vi "Locate.vi"() -> ()   [LabVIEW 2017]
uses:
  <vilib>/Utility/file.llb/Write Delimited Spreadsheet (DBL).vi
  <vilib>/vision/driver/NI_Vision_Acquisition_Software.lvlib
  <vilib>/vision/NI_Vision_Development_Module.lvlib
panel:
  out "Boolean 2":bool
  out "X":dbl[](array[numeric])
  out "Numeric 2":dbl
  out "Numeric":dbl
  out "OK Y":dbl
  out "OK X":dbl
  in  "OK Button":bool
  out "Boolean":bool
  out "Y":dbl[](array[numeric])
  out "選擇範圍 2":T1(plugin-control)
  out "error out":errorcluster
  in  "亮度":cluster{"Min":i32, "Max":i32}(slide)={"Min"=60, "Max"=157} scale=0.0..255.0
  in  "飽和度":cluster{"Min":i32, "Max":i32}(slide)={"Min"=0, "Max"=42} scale=0.0..255.0
  in  "色相":cluster{"Min":i32, "Max":i32}(slide)={"Min"=67, "Max"=120} scale=0.0..255.0
  out "顯示錯誤":errorcluster
  out "影像":T1(plugin-control)
  in  "stop":bool
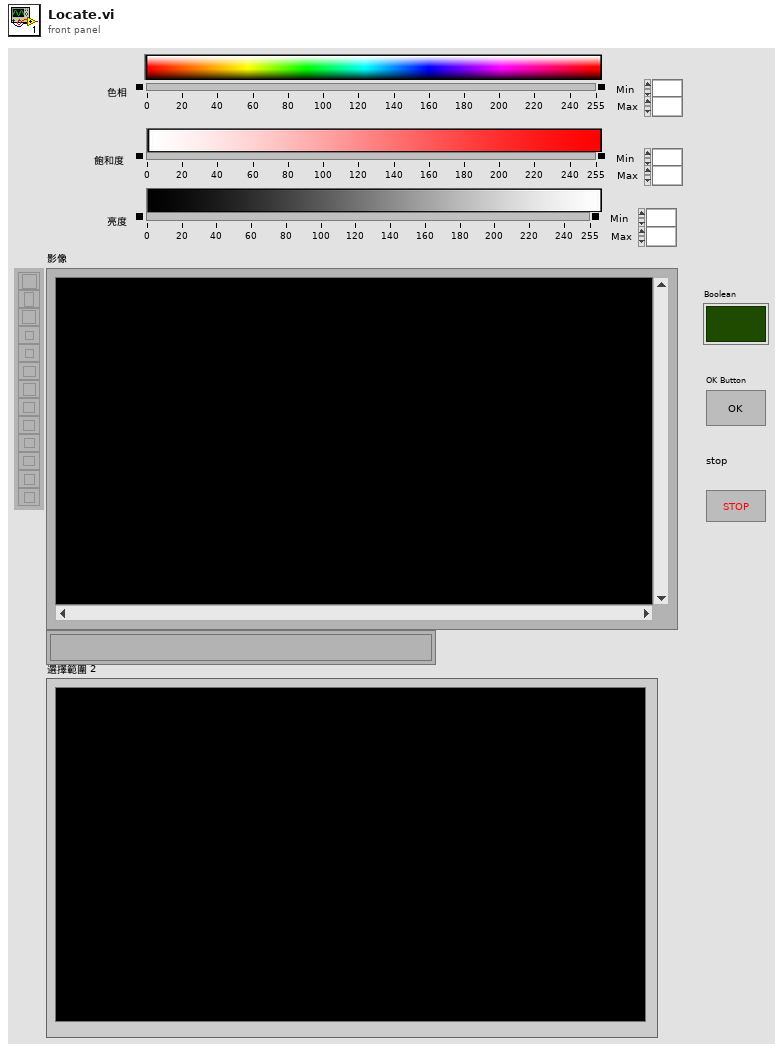
[diagram p1: front panel]
types:
  T1 = typedef "IMAQ Image.ctl" = refnum<image>
  T2 = typedef "Image Type" = u32
  T3 = cluster{"Type":u32, "Version":u32, "Flags":u32, "SerialNumberHigh":u32, "SerialNumberLow":u32, "BusType":u32, "InterfaceName":string, "VendorName":string, "ModelName":string, "CameraFileName":string, "CameraAttributeURL":string}[]
  T4 = cluster{"Type":u32, "Version":u32, "Flags":u32, "SerialNumberHigh":u32, "SerialNumberLow":u32, "BusType":u32, "InterfaceName":string, "VendorName":string, "ModelName":string, "CameraFileName":string, "CameraAttributeURL":string}
  T5 = typedef "IMAQdx.ctl" = refnum<k21>
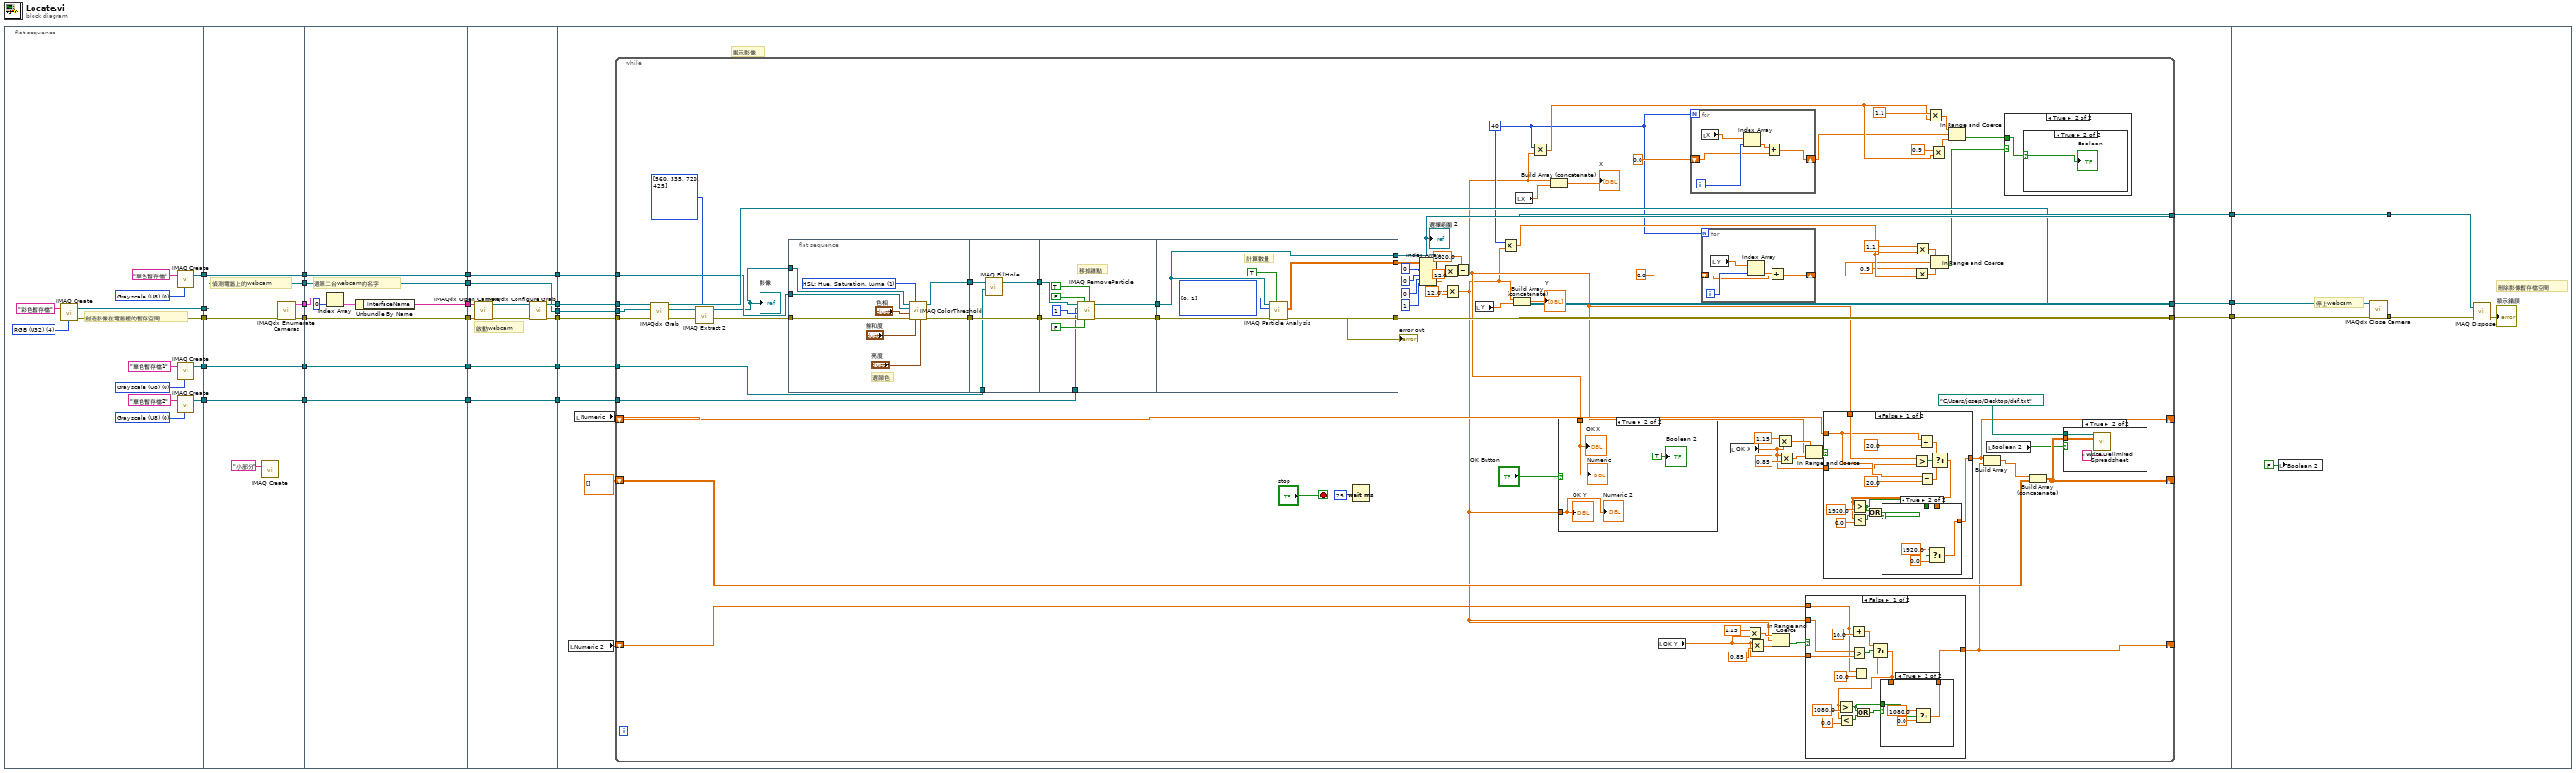
[diagram p0: block diagram]
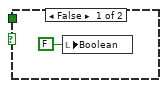
[diagram p3: hidden frame]
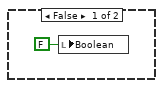
[diagram p4: hidden frame]
diagram:
  n1 = flat-sequence {
    tunnel: [w39] -> w22
    tunnel: [w38] -> w21
    tunnel: [w35] -> w12
    tunnel: [w30] -> w5
    tunnel: [w29] -> w1
    tunnel: [w49] -> w28
    tunnel: [w48] -> w23
    tunnel: w22 -> [w48]
    tunnel: w21 -> [w47]
    tunnel: [w46] -> w19
    tunnel: [w45] -> w13
    tunnel: w12 -> [w45]
    tunnel: [w44] -> w6
    tunnel: w5 -> [w44]
    tunnel: [w43] -> w2
    tunnel: w1 -> [w43]
    tunnel: w28 -> [w56]
    tunnel: [w55] -> w27
    tunnel: [w54] -> w24
    tunnel: w23 -> [w54]
    tunnel: [w53] -> w20
    tunnel: w19 -> [w53]
    tunnel: [w52] -> w14
    tunnel: w13 -> [w52]
    tunnel: [w51] -> w7
    tunnel: w6 -> [w51]
    tunnel: [w50] -> w3
    tunnel: w2 -> [w50]
    tunnel: w27 -> [w67]
    tunnel: [w66] -> w26
    tunnel: [w65] -> w25
    tunnel: w24 -> [w65]
    tunnel: w20 -> [w64]
    tunnel: [w62] -> w18
    tunnel: [w61] -> w15
    tunnel: w14 -> [w61]
    tunnel: [w60] -> w8
    tunnel: w7 -> [w60]
    tunnel: [w59] -> w4
    tunnel: w3 -> [w59]
    tunnel: w26 -> [w80]
    tunnel: w25 -> [w79]
    tunnel: w18 -> [w78]
    tunnel: [w77] -> w16
    tunnel: w15 -> [w76]
    tunnel: [w75] -> w11
    tunnel: [w74] -> w10
    tunnel: w8 -> [w73]
    tunnel: w4 -> [w72]
    tunnel: [w252] -> w17
    tunnel: w16 -> [w251]
    tunnel: w11 -> [w250]
    tunnel: w10 -> [w249]
    tunnel: [w249] -> w9
    tunnel: w17 -> [w255]
    tunnel: w9 -> [w253]
    frame #0 {
      w33 = T2 0 items=["Grayscale (U8)", "Grayscale (I16)", "Grayscale (SGL)", "Complex (CSG)", "RGB (U32)", "HSL (U32)", "RGB (U64)", "Grayscale (U16)"] ("Image Type")
      w34 = T2 0 items=["Grayscale (U8)", "Grayscale (I16)", "Grayscale (SGL)", "Complex (CSG)", "RGB (U32)", "HSL (U32)", "RGB (U64)", "Grayscale (U16)"] ("Image Type")
      w36 = T2 0 items=["Grayscale (U8)", "Grayscale (I16)", "Grayscale (SGL)", "Complex (CSG)", "RGB (U32)", "HSL (U32)", "RGB (U64)", "Grayscale (U16)"] ("Image Type")
      w41 = T2 4 items=["Grayscale (U8)", "Grayscale (I16)", "Grayscale (SGL)", "Complex (CSG)", "RGB (U32)", "HSL (U32)", "RGB (U64)", "Grayscale (U16)"] ("Image Type")
      # "創造影像在電腦裡的暫存空間"
      n2 = call "IMAQ Create"("Image Name"="彩色暫存檔", "Image Type"=w41) -> ("New Image"=w39:T1, "error out"=w38:errorcluster)  [unwired: 3 in]
      n3 = call "IMAQ Create"("Image Name"="單色暫存檔", "Image Type"=w36) -> ("New Image"=w35:T1)  [unwired: 3 in, 1 out]
      n4 = call "IMAQ Create"("Image Name"="單色暫存檔1", "Image Type"=w34) -> ("New Image"=w30:T1)  [unwired: 3 in, 1 out]
      n5 = call "IMAQ Create"("Image Name"="單色暫存檔2", "Image Type"=w33) -> ("New Image"=w29:T1)  [unwired: 3 in, 1 out]
    }
    frame #1 {
      # "偵測電腦上的webcam"
      n6 = call "IMAQ Create"("Image Name"="小部分") -> ()  [unwired: 4 in, 2 out]
      n7 = call <vilib>:"IMAQdx Enumerate Cameras.vi"("error in"=w47) -> ("error out"=w46:errorcluster, "Camera Information Array"=w49:T3)  [unwired: 9 in]
    }
    frame #2 {
      # "選第二台webcam的名字"
      n8 = Index Array(array=w56, index=0) -> (element=w57:T4)
      n9 = Unbundle By Name(w57) -> ("InterfaceName"=w55:string)
    }
    frame #3 {
      # "啟動webcam"
      n10 = call <vilib>:"IMAQdx Open Camera.vi"("error in"=w64, "Session In"=w67) -> ("error out"=w63:errorcluster, "Session Out"=w68:T5)  [unwired: 8 in]
      n11 = call <vilib>:"IMAQdx Configure Grab.vi"("error in"=w63, "Session In"=w68) -> ("error out"=w62:errorcluster, "Session Out"=w66:T5)  [unwired: 8 in]
    }
    frame #4 {
      # "顯示影像"
      n12 = local read "Numeric 2"() -> (w70:dbl)
      n13 = local read "Numeric"() -> (w71:dbl)
      n14 = while {
        tunnel: w80 -> [w156]
        tunnel: w79 -> [w92]
        tunnel: w78 -> [w155]
        tunnel: [w154] -> w77
        tunnel: w76 -> [w143]
        tunnel: [w145] -> w75
        tunnel: [w144] -> w74
        tunnel: w73 -> [w138]
        tunnel: w72 -> [w137]
        shift-right: [w93] -> _
        shift-left: w71 -> [w119]
        shift-right: [w94] -> _
        shift-left: w70 -> [w108]
        shift-right: [w109] -> _
        shift-left: dbl[][] [] -> [w110]
        stop <- "stop" stop-if-true
        w88 = 40
        n15 = call <vilib>:"IMAQdx Grab.vi"("error in"=w155, "Image In"=w92, "Session In"=w156) -> ("error out"=w147:errorcluster, "Image Out"=w91:T1, "Session Out"=w154:T5)  [unwired: 5 in, 1 out]
        n16 = call "IMAQ Extract 2"("Optional Rectangle"=i32[] [560, 335, 720, 425], "Image Src"=w91) -> ("Image Dst Out"=w90:T1)  [unwired: 8 in, 1 out]
        "影像" <- w90
        n17 = flat-sequence {
          tunnel: w147 -> [w222]
          tunnel: w90 -> [w224]
          tunnel: [w221] -> w141
          tunnel: w143 -> [w223]
          tunnel: [w220] -> w139
          tunnel: [w230] -> w142
          tunnel: w141 -> [w232]
          tunnel: [w232] -> w140
          tunnel: w139 -> [w231]
          tunnel: w138 -> [w229]
          tunnel: [w235] -> w149
          tunnel: [w234] -> w148
          tunnel: w142 -> [w237]
          tunnel: w140 -> [w236]
          tunnel: w137 -> [w233]
          tunnel: [w246] -> w144
          tunnel: [w242] -> w145
          tunnel: w149 -> [w245]
          tunnel: w148 -> [w246]
          tunnel: [w243] -> w146
          frame #0 {
            w225 = 1 items=["RGB (Red, Green, Blue)", "HSL: Hue, Saturation, Luma"] ("Threshold Color Mode")
            # "選顏色"
            n18 = call "IMAQ ColorThreshold"("Blue or Luma or Val or Inten Range"="亮度", "Green or Sat Range"="飽和度", "Color Mode"=w225, "error in (no error)"=w222, "Red or Hue Range"="色相", "Image Dst"=w223, "Image Src"=w224) -> ("error out"=w221:errorcluster, "Image Dst Out"=w220:T1)  [unwired: 1 in, 2 out]
          }
          frame #1 {
            n19 = call "IMAQ FillHole"("Image Dst"=w229, "Image Src"=w231) -> ("Image Dst Out"=w230:T1)  [unwired: 2 in, 3 out]
          }
          frame #2 {
            # "移掉雜點"
            n20 = call "IMAQ RemoveParticle"("Connectivity 4/8 (8)"=TRUE, "Low Pass/High Pass (Low)"=FALSE, "Square/Hexa (Square)"=FALSE, "error in (no error)"=w236, "Number of Erosion"=1, "Image Dst"=w233, "Image Src"=w237) -> ("error out"=w235:errorcluster, "Image Dst Out"=w234:T1)  [unwired: 3 out]
          }
          frame #3 {
            w244 = i32[] [0, 1] items=["Center of Mass X", "Center of Mass Y", "First Pixel X", "First Pixel Y", "Bounding Rect Left", "Bounding Rect Top", "Bounding Rect Right", "Bounding Rect Bottom", "Max Feret Diameter Start X", "Max Feret Diameter Start Y", "Max Feret Diameter End X", "Max Feret Diameter End Y", "Max Horiz. Segment Length Left", "Max Horiz. Segment Length Right", "Max Horiz. Segment Length Row", "-", "Bounding Rect Width", "Bounding Rect Height", "Bounding Rect Diagonal", "Perimeter", "Convex Hull Perimeter", "Holes' Perimeter", "Max Feret Diameter", "Equivalent Ellipse Major Axis", "Equivalent Ellipse Minor Axis", "Equivalent Ellipse Minor Axis (Feret)", "Equivalent Rect Long Side", "Equivalent Rect Short Side", "Equivalent Rect Diagonal", "Equivalent Rect Short Side (Feret)", "Average Horiz. Segment Length", "Average Vert. Segment Length", "Hydraulic Radius", "Waddel Disk Diameter", "-", "Area", "Holes' Area", "Particle & Holes' Area", "Convex Hull Area", "Image Area", "-", "Number of Holes", "Number of Horiz. Segments", "Number of Vert. Segments", "-", "Orientation", "Max Feret Diameter Orientation", "-", "% Area/Image Area", "% Area/(Particle & Holes' Area)", "Ratio of Equivalent Ellipse Axes", "Ratio of Equivalent Rect Sides", "-", "Elongation Factor", "Compactness Factor", "Heywood Circularity Factor", "Type Factor", "-", "Sum X", "Sum Y", "Sum XX", "Sum XY", "Sum YY", "Sum XXX", "Sum XXY", "Sum XYY", "Sum YYY", "-", "Moment of Inertia XX", "Moment of Inertia XY", "Moment of Inertia YY", "Moment of Inertia XXX", "Moment of Inertia XXY", "Moment of Inertia XYY", "Moment of Inertia YYY", "Norm. Moment of Inertia XX", "Norm. Moment of Inertia XY", "Norm. Moment of Inertia YY", "Norm. Moment of Inertia XXX", "Norm. Moment of Inertia XXY", "Norm. Moment of Inertia XYY", "Norm. Moment of Inertia YYY", "Hu Moment 1", "Hu Moment 2", "Hu Moment 3", "Hu Moment 4", "Hu Moment 5", "Hu Moment 6", "Hu Moment 7"] ("Pixel Measurements")
            # "計算數量"
            n21 = call "IMAQ Particle Analysis"("Connectivity 4/8 (8)"=TRUE, "error in (no error)"=w245, "Pixel Measurements"=w244, "Image"=w246) -> ("error out"=w242:errorcluster, "Particle Measurements (Pixels)"=w243:dbl[][])  [unwired: 1 in, 5 out]
          }
        }
        n22 = Wait (ms)(milliseconds to wait=u32 25 ("millisecond timer value")) -> ()  [unwired: 1 out]
        n23 = Index Array(array=w146, index (row) #1=0 ("disabled index (row)"), index (col) #1=0 ("disabled index (col)"), index (row) #2=0 ("index (row)"), index (col) #2=1 ("disabled index (col)")) -> (element #1=w104:dbl, element #2=w107:dbl)
        n24 = Multiply(x=w104, y=12.0) -> (x*y=w87:dbl)
        n25 = Multiply(x=12.0, y=w107) -> (x*y=w81:dbl)
        n26 = Subtract(x=1920.0, y=w87) -> (x-y=w83:dbl)
        n27 = local read "Y"() -> (w135:dbl[])
        n28 = Multiply(x=w88, y=w81) -> (x*y=w130:dbl)
        n29 = Build Array (concatenate)(w81, w135) -> (→"Y":dbl[])
        n30 = local read "X"() -> (w105:dbl[])
        n31 = Multiply(x=w88, y=w83) -> (x*y=w98:dbl)
        n32 = Build Array (concatenate)(w83, w105) -> (→"X":dbl[])
        n33 = case shown="True" "OK Button" {
          tunnel: w83 -> [_ w213]
          tunnel: w81 -> [_ w214]
          frame False {
          }
          frame True {
            "OK X" <- w213
            "OK Y" <- w214
            "Numeric" <- w213
            "Numeric 2" <- w214
            "Boolean 2" <- TRUE ("Boolean 2")
          }
        }
        n34 = local read "OK Y"() -> (w112:dbl)
        n35 = for {
          N: w88 -> [_]
          shift-right: [w166] -> w97
          shift-left: 0.0 -> [w165]
          i -> [w168]
          n36 = local read "X"() -> (w169:dbl[])
          n37 = Index Array(array=w169, index=w168) -> (element=w167:dbl)
          n38 = Add(x=w167, y=w165) -> (x+y=w166:dbl)
        }
        n39 = for {
          N: w88 -> [_]
          shift-right: [w216] -> w129
          shift-left: 0.0 -> [w215]
          i -> [w218]
          n40 = local read "Y"() -> (w219:dbl[])
          n41 = Index Array(array=w219, index=w218) -> (element=w217:dbl)
          n42 = Add(x=w217, y=w215) -> (x+y=w216:dbl)
        }
        n43 = local read "OK X"() -> (w118:dbl)
        n44 = Multiply(x=1.15, y=w112) -> (x*y=w116:dbl)
        n45 = Multiply(x=w112, y=0.85) -> (x*y=w115:dbl)
        n46 = In Range and Coerce(upper limit=w116, x=w81, lower limit=w115) -> (In Range?=w117:bool)  [unwired: 1 out]
        n47 = Multiply(x=1.15, y=w118) -> (x*y=w121:dbl)
        n48 = Multiply(x=w118, y=0.85) -> (x*y=w120:dbl)
        n49 = In Range and Coerce(upper limit=w121, x=w83, lower limit=w120) -> (In Range?=w124:bool)  [unwired: 1 out]
        n50 = case shown="False" w117 {
          tunnel: [w171 w190] -> w94
          tunnel: w112 -> [w179 _]
          tunnel: w81 -> [w178 w190]
          tunnel: w108 -> [w177 _]
          frame False {
            n51 = Add(x=w177, y=10.0) -> (x+y=w184:dbl)
            n52 = Greater?(x=w178, y=w179) -> (0:w180:bool)
            n53 = Subtract(x=w177, y=10.0) -> (x-y=w183:dbl)
            n54 = Select(t=w184, s=w180, f=w183) -> (s? t:f=w170:dbl)
            n55 = Greater?(x=w170, y=1080.0) -> (0:w172:bool)
            n56 = Less?(x=w170, y=0.0) -> (x < y?=w175:bool)
            n57 = Or(x=w172, y=w175) -> (x .or. y?=w176:bool)
            n58 = case shown="True" w176 {
              tunnel: w172 -> [_ w189]
              tunnel: w170 -> [w185 _]
              tunnel: [w185 w186] -> w171
              frame False {
              }
              frame True {
                n59 = Select(t=1080.0, s=w189, f=0.0) -> (s? t:f=w186:dbl)
              }
            }
          }
          frame True {
          }
        }
        n60 = case shown="False" w124 {
          tunnel: [w193 w211] -> w93
          tunnel: w83 -> [w204 _]
          tunnel: w119 -> [w199 w211]
          tunnel: w118 -> [w198 _]
          frame False {
            n61 = Greater?(x=w204, y=w198) -> (0:w205:bool)
            n62 = Add(x=w199, y=20.0) -> (x+y=w200:dbl)
            n63 = Subtract(x=w199, y=20.0) -> (x-y=w201:dbl)
            n64 = Select(t=w200, s=w205, f=w201) -> (s? t:f=w191:dbl)
            n65 = Greater?(x=w191, y=1920.0) -> (0:w192:bool)
            n66 = Less?(x=w191, y=0.0) -> (x < y?=w197:bool)
            n67 = Or(x=w192, y=w197) -> (x .or. y?=w194:bool)
            n68 = case shown="True" w194 {
              tunnel: [w206 w207] -> w193
              tunnel: w191 -> [w206 _]
              tunnel: w192 -> [_ w210]
              frame False {
              }
              frame True {
                n69 = Select(t=1920.0, s=w210, f=0.0) -> (s? t:f=w207:dbl)
              }
            }
          }
          frame True {
          }
        }
        n70 = Multiply(x=0.9, y=w130) -> (x*y=w131:dbl)
        n71 = Multiply(x=1.1, y=w130) -> (x*y=w132:dbl)
        n72 = Multiply(x=1.1, y=w98) -> (x*y=w102:dbl)
        n73 = Multiply(x=0.9, y=w98) -> (x*y=w101:dbl)
        n74 = In Range and Coerce(upper limit=w132, x=w129, lower limit=w131) -> (In Range?=w96:bool)  [unwired: 1 out]
        n75 = In Range and Coerce(upper limit=w102, x=w97, lower limit=w101) -> (In Range?=w95:bool)  [unwired: 1 out]
        n76 = Build Array(w93, w94) -> (w111:dbl[])
        n77 = local read "Boolean 2"() -> (w84:bool)
        n78 = case shown="True" w96 {
          tunnel: w95 -> [_ w162]
          frame False {
            n79 = local write "Boolean"(FALSE ("Boolean")) -> ()
          }
          frame True {
            n80 = case shown="True" w162 {
              selector: w162 -> [_ w164]
              frame False {
                n81 = local write "Boolean"(FALSE ("Boolean")) -> ()
              }
              frame True {
                "Boolean" <- w164
              }
            }
          }
        }
        n82 = Build Array (concatenate)(w111, w110) -> (w109:dbl[][])
        n83 = case shown="True" w84 {
          tunnel: path "C:/Users/josep/Desktop/def.txt" ("file path (dialog if empty)") -> [_ w160]
          tunnel: w109 -> [_ w159]
          frame False {
          }
          frame True {
            n84 = call-poly <vilib>:"Write Delimited Spreadsheet.vi"("file path (dialog if empty)"=w160, "2D data"=w159, "delimiter (\\t)"=" " ("delimiter (\\t)")) -> ()  [unwired: 11 in, 2 out]
          }
        }
        "error out" <- w145
        "選擇範圍 2" <- w144
      }
    }
    frame #5 {
      # "停止webcam"
      n85 = local write "Boolean 2"(FALSE ("Boolean 2")) -> ()
      n86 = call <vilib>:"IMAQdx Close Camera.vi"("error in"=w250, "Session In"=w251) -> ("error out"=w252:errorcluster)  [unwired: 9 in]
    }
    frame #6 {
      # "刪除影像暫存檔空間"
      n87 = call "IMAQ Dispose"("Image"=w253, "error in (no error)"=w255) -> ("error out"=→"顯示錯誤":errorcluster)  [unwired: 4 in]
    }
  }
